vi "BRAM_ReadVITLogo.vi"(2 "Address":i16) -> (16 "PixelData":bool[](array[boolean]))   [LabVIEW 2018]
uses:
  <vilib>/rvi/Memory/Memory_Emulation/nirvimemoryFastEmulation.vi
  <vilib>/rvi/Memory/Memory_Emulation/nirvimemoryEmulation.vi
  <vilib>/rvi/Emulation/niFpgaEmulationIsFPGAContextNoSignature.vi
  <vilib>/rvi/DataTransferAndStorage/Container/Common/niFpgaContainerGetUniqueNameForEmu.vi
  <vilib>/rvi/Emulation/niFpgaProcessEmulError.vi
  <vilib>/rvi/Emulation/niFpgaSctlEmulationGetInTimedLoop.vi
  <vilib>/rvi/errors/nirviReportUnexpectedCaseInternalError (U32).vi
  <vilib>/rvi/DataTransferAndStorage/Container/XNode/niFpgaContainer.xnode
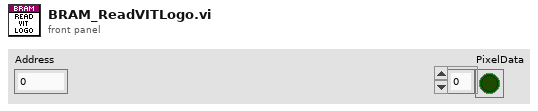
[diagram p1: front panel]
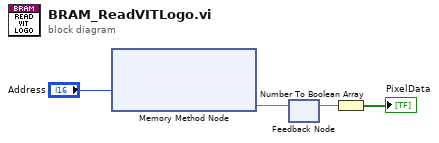
[diagram p0: block diagram]
diagram:
  n1 = xnode ("Memory Method Node")("Address A"="Address") -> ("Data A"=w3:fxp<+,12,12>)  [unwired: 1 in, 1 out]
  n2 = feedback-in #1(w3) -> ()
  n3 = feedback #1() -> (w2:fxp<+,12,12>)  [unwired: 1 in]
  n4 = Number To Boolean Array(number=w2) -> (Boolean array=→"PixelData":bool[])
